vi "Get XC Report.vi"(9 "timeout in ms (60000)":i32=60000, 10 "selected path":path, 11 "HPS-17000 in":refnum<class "HPS-17000.lvclass">) -> (0 "error out":errorcluster, 3 "HPS-17000 out":refnum<class "HPS-17000.lvclass">)   [LabVIEW 2023]
uses:
  <instrlib>/HPS-17000/HPS-17000.lvclass
  <instrlib>/HPS-17000/Internal/Get Diagnostic Data Single.vi
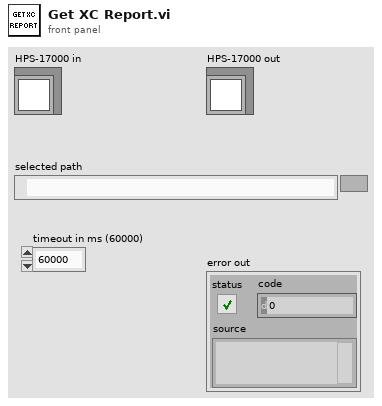
[diagram p1: front panel]
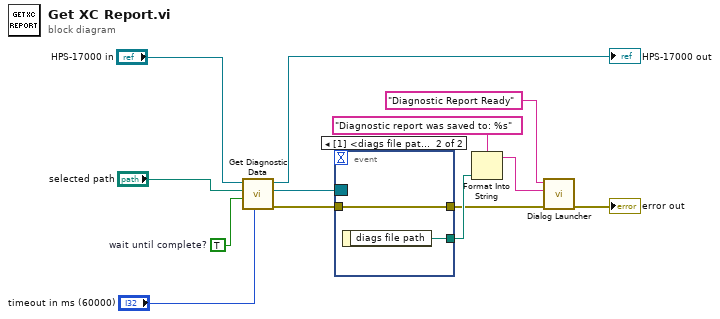
[diagram p0: block diagram]
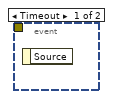
[diagram p2: hidden frame]
diagram:
  w3 = TRUE  # wait until complete?
  n1 = call-poly <instrlib>:"Get Diagnostic Data.vi"("timeout in ms (60000)"="timeout in ms (60000)", "wait until complete?"=w3, "destination path"="selected path", "HPS-17000 in"="HPS-17000 in") -> ("error out"=w7:errorcluster, "file ready event registration"=w6:refnum<event-registration>, "HPS-17000 out"=→"HPS-17000 out":refnum<class "HPS-17000.lvclass">)  [unwired: 5 in]
  n2 = event shown="[1] <diags file path>: User Event" {
    selector: w6 -> [_ _]
    dyn-events: _ -> [_ _]
    timeout: _ -> [_ _]
    tunnel: w7 -> [_ w15]
    tunnel: [_ w15] -> w8
    tunnel: [_ w14] -> w11
    event Timeout {
      n3 = event-data() -> ()  [unwired: 1 in, 1 out]
    }
    event User Event {
      n4 = event-data() -> ("diags file path"=w14:path)  [unwired: 1 in]
    }
  }
  n5 = Format Into String(format string="Diagnostic report was saved to: %s", w11) -> (resulting string=w12:string)  [unwired: 2 in, 1 out]
  n6 = call "Dialog Launcher.vi"("error in (no error)"=w8, "Message"=w12, "Title"="Diagnostic Report Ready") -> ("error out"=→"error out":errorcluster)  [unwired: 8 in]
